vi "多参校准.vi"   [LabVIEW 2016, in "斯坦道仪器.lvlib"]
uses:
  PLC/PLC.lvlib
types:
  T1 = cluster{"starting address":u16, "holding register value":u16}
  T2 = enum16{"idle", "init", "读状态", "读参数", "多个写入", "单个写入", "线圈写入"}
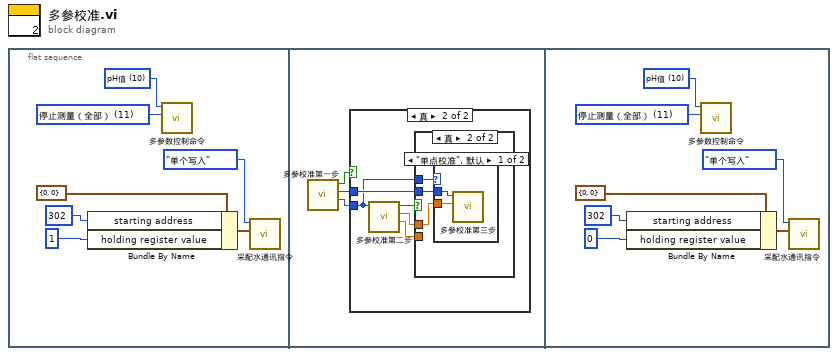
[diagram p0: block diagram]
diagram:
  n1 = flat-sequence {
    frame #0 {
      w1 = u16 11 items=["启动测量（全部）"=1, "初始化（清洗）"=10, "停止测量（全部）"=11, "校时"=13, "启动测量（单个传感器）"=19, "停止测量（单个传感器）"=20] ("控制命令")
      w2 = u16 10 items=["氨氮"=3, "水温"=9, "pH值"=10, "溶解氧"=11, "电导率"=12, "浊度"=13, "叶绿素a"=14, "藻密度"=15, "蓝绿藻"=16, "氧化还原电位"=17, "溶解氧%"=18, "盐度"=19] ("站号")
      n2 = Bundle By Name(cluster=T1 {"starting address"=0, "holding register value"=0}, "starting address"=u16 302, "holding register value"=u16 1) -> (w5:T1)
      n3 = call "多参数控制命令.vi"("控制命令"=w1, "站号"=w2) -> ()  [unwired: 9 in, 1 out]
      n4 = call "采配水通讯指令.vi"("数据"=w5, "命令"=T2."单个写入") -> ()  [unwired: 10 in]
    }
    frame #1 {
      n5 = call "多参校准第一步.vi"() -> ("校准模式选择"=w8:enum32{"单点校准", "多点校准"}, "校准探头"=w9:u16, "继续执行"=w10:bool)  [unwired: 9 in]
      n6 = case shown="真" w10 {
        tunnel: w9 -> [_ w13]
        tunnel: w8 -> [_ w12]
        frame False {
        }
        frame True {
          n7 = call "多参校准第二步.vi"("校准模式"=w12) -> ("标样2浓度输出"=w11:dbl, "标样1浓度输出"=w14:dbl, "继续执行"=w15:bool)  [unwired: 8 in]
          n8 = case shown="真" w15 {
            tunnel: w14 -> [_ w17]
            tunnel: w13 -> [_ w18]
            tunnel: w12 -> [_ w16]
            tunnel: w11 -> [_ _]
            frame False {
            }
            frame True {
              n9 = case shown="\"单点校准\", 默认" w16 {
                tunnel: w18 -> [w20 _]
                tunnel: w17 -> [w19 _]
                frame "单点校准", Default {
                  n10 = call "多参校准第三步.vi"("标样1浓度输出"=w19, "探头选择"=w20) -> ()  [unwired: 8 in, 2 out]
                }
                frame "多点校准" {
                }
              }
            }
          }
        }
      }
    }
    frame #2 {
      w22 = u16 11 items=["启动测量（全部）"=1, "初始化（清洗）"=10, "停止测量（全部）"=11, "校时"=13, "启动测量（单个传感器）"=19, "停止测量（单个传感器）"=20] ("控制命令")
      w21 = u16 10 items=["氨氮"=3, "水温"=9, "pH值"=10, "溶解氧"=11, "电导率"=12, "浊度"=13, "叶绿素a"=14, "藻密度"=15, "蓝绿藻"=16, "氧化还原电位"=17, "溶解氧%"=18, "盐度"=19] ("站号")
      n11 = Bundle By Name(cluster=T1 {"starting address"=0, "holding register value"=0}, "starting address"=u16 302, "holding register value"=u16 0) -> (w25:T1)
      n12 = call "多参数控制命令.vi"("控制命令"=w22, "站号"=w21) -> ()  [unwired: 9 in, 1 out]
      n13 = call "采配水通讯指令.vi"("数据"=w25, "命令"=T2."单个写入") -> ()  [unwired: 10 in]
    }
  }
